vi "Euc_distance.vi"(10 "Centroid":dbl[](array[numeric]), 11 "Values (row = members, \ncolumn = sample Num)":dbl[](array[numeric])) -> (3 "Euclidean\nDistance":dbl)   [LabVIEW 2014]
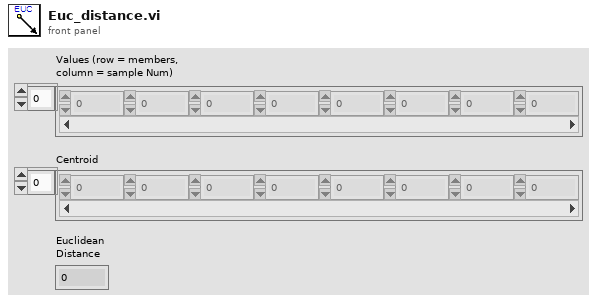
[diagram p1: front panel]
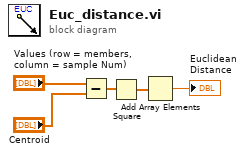
[diagram p0: block diagram]
diagram:
  n1 = Subtract(x="Values (row = members, \ncolumn = sample Num)", y="Centroid") -> (x-y=w4:dbl[])
  n2 = Square(x=w4) -> (x^2=w5:dbl[])
  n3 = Add Array Elements(numeric array=w5) -> (sum=→"Euclidean\nDistance":dbl)
